vi "Core_[HSMS]Not Selected(Active).vi"(8 "error in (no error)":errorcluster, 11 "HSMS Class in":refnum<class "HSMS Class.lvclass">) -> (0 "error out":errorcluster, 3 "HSMS Class out":refnum<class "HSMS Class.lvclass">)   [LabVIEW 2020, in "SECS Communication.lvlib" / "HSMS Class.lvclass"]
uses:
  HSMS Class.lvclass
  SType.ctl
  Message Packet.ctl
  Message Header.ctl
  PType.ctl
  Notifier Type.ctl
  HSMS Class.lvclass/HSMS Class.ctl
  HSMS State.ctl
  Read Session ID.vi
  Read T6(Control Timeout).vi
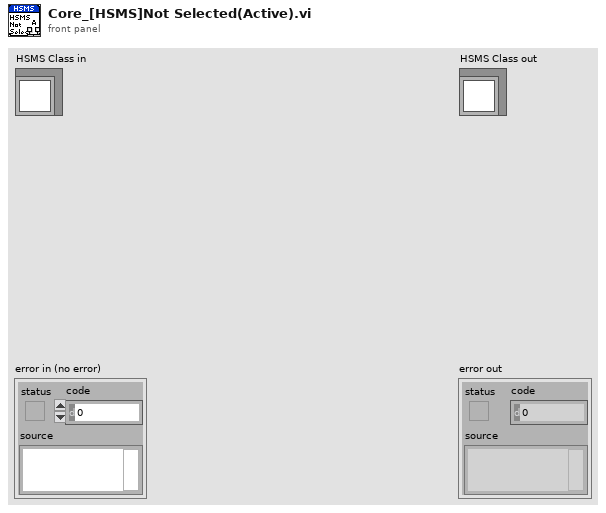
[diagram p1: front panel]
types:
  T1 = typedef "SECS Communication.lvlib/HSMS Class.lvclass/Message Header.ctl" = cluster{"Byte 0-1(Session ID)":u16, "W-Bit":bool, "Byte 2":u8, "Byte 3":u8, "Byte 4(PType)":T2, "Byte 5(SType)":T3, "Byte 6-9(System Btyes)":u8[]}
  T2 = typedef "SECS Communication.lvlib/HSMS Class.lvclass/PType.ctl" = enum8{"SECS-II Encoding", "Reserved"}
  T3 = typedef "SECS Communication.lvlib/HSMS Class.lvclass/SType.ctl" = enum8{"Data Message", "Select.req", "Select.rsp", "Deselect.req", "Deselect.rsp", "Linktest.req", "Linktest.rsp", "Reject.req", "Separate.req"}
  T4 = typedef "SECS Communication.lvlib/HSMS Class.lvclass/Notifier Type.ctl" = enum16{"TCPIP Connect", "TCPIP Disconnect", "Receive Message", "Send Message", "T3 Timeout", "T6 Timeout", "T7 Timeout", "Error", "Stop"}
  T5 = typedef "SECS Communication.lvlib/HSMS Class.lvclass/Message Packet.ctl" = cluster{"Message Header Cluster":T1, "Message Header":u8[], "Message Text":u8[]}
  T6 = typedef "SECS Communication.lvlib/HSMS Class.lvclass/HSMS State.ctl" = enum16{"[TCP/IP]Not Connect", "[HSMS]Not Selected", "[HSMS]Selected", "Stop"}
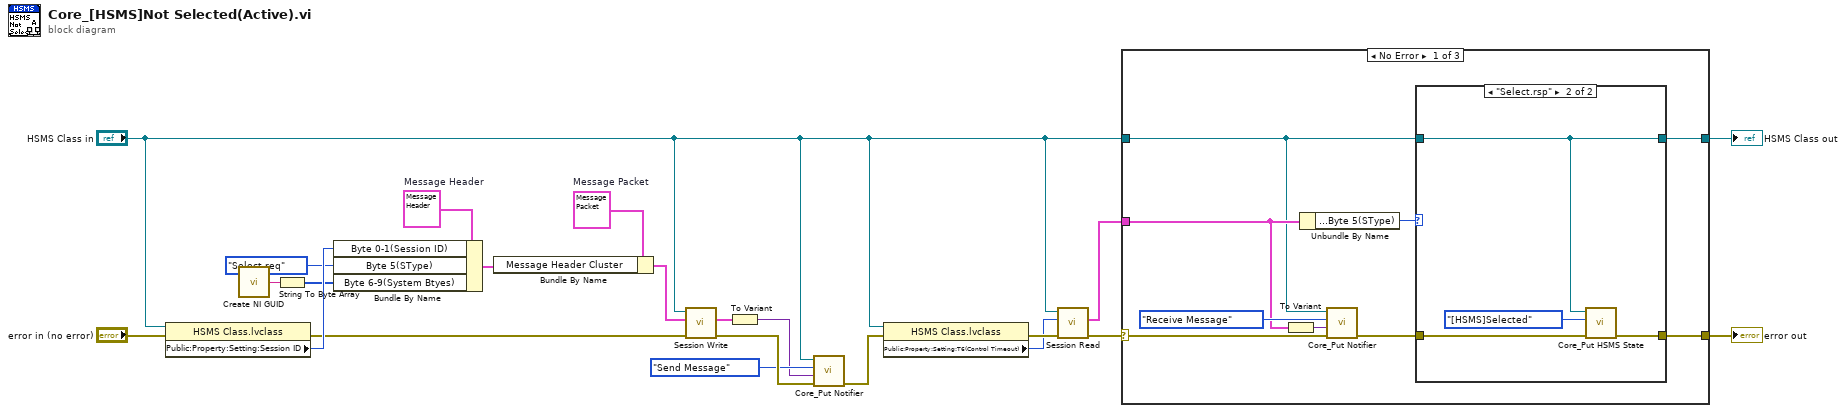
[diagram p0: block diagram]
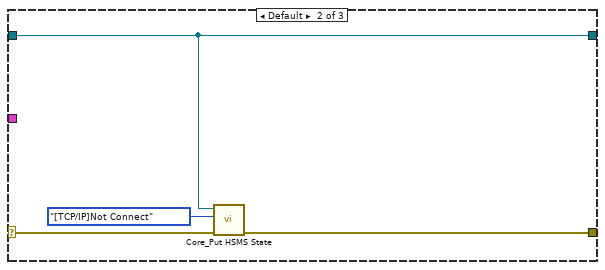
[diagram p3: hidden frame]
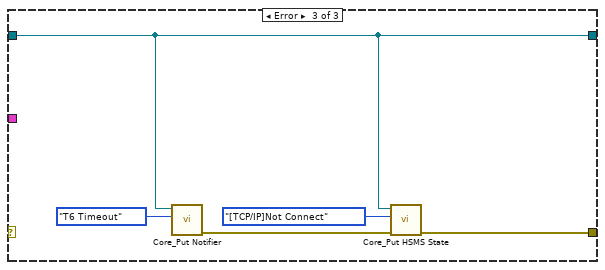
[diagram p4: hidden frame]
diagram:
  w18 = T1 {"Byte 0-1(Session ID)"=0, "W-Bit"=FALSE, "Byte 2"=0, "Byte 3"=0, "Byte 4(PType)"=enum."SECS-II Encoding", "Byte 5(SType)"=enum."Select.req", "Byte 6-9(System Btyes)"=[]}  # Message Header
  w13 = T5 {"Message Header Cluster"={"Byte 0-1(Session ID)"=0, "W-Bit"=FALSE, "Byte 2"=0, "Byte 3"=0, "Byte 4(PType)"=enum."SECS-II Encoding", "Byte 5(SType)"=enum."Data Message", "Byte 6-9(System Btyes)"=[]}, "Message Header"=[], "Message Text"=[]}  # Message Packet
  n1 = property class="HSMS Class.lvclass"(reference="HSMS Class in", error in="error in (no error)") -> (error out=w9:errorcluster, "Public:Property:Setting:Session ID"=w17:u16)  [unwired: 1 out]
  n2 = call <vilib>:"Create NI GUID.vi"() -> ("NI GUID"=w15:string)
  n3 = String To Byte Array(string=w15) -> (unsigned byte array=w14:u8[])
  n4 = Bundle By Name(cluster=w18, "Byte 0-1(Session ID)"=w17, "Byte 5(SType)"=SType."Select.req", "Byte 6-9(System Btyes)"=w14) -> (w12:T1)
  n5 = Bundle By Name(cluster=w13, "Message Header Cluster"=w12) -> (w6:T5)
  n6 = call "Session Write.vi"("error in (no error)"=w9, "Message Packet In"=w6, "HSMS Class in"="HSMS Class in") -> ("error out"=w8:errorcluster, "Message Packet Out"=w1:T5)  [unwired: 6 in, 1 out]
  n7 = To Variant(anything=w1) -> (Variant=w5:variant)
  n8 = call "Core_Put Notifier.vi"("error in (no error)"=w8, "Data"=w5, "Notifier Type"=Notifier_Type."Send Message", "HSMS Class in"="HSMS Class in") -> ("error out"=w4:errorcluster)  [unwired: 6 in, 1 out]
  n9 = property class="HSMS Class.lvclass"(reference="HSMS Class in", error in=w4) -> (error out=w3:errorcluster, "Public:Property:Setting:T6(Control Timeout)"=w2:i32)  [unwired: 1 out]
  n10 = call "Session Read.vi"("error in (no error)"=w3, "Timeout"=w2, "HSMS Class in"="HSMS Class in") -> ("error out"=w10:errorcluster, "Message Packet"=w11:T5)  [unwired: 6 in, 1 out]
  n11 = case shown="No Error" w10 {
    selector: w10 -> [w28 w40 _]
    tunnel: w11 -> [w27 _ _]
    tunnel: [w30 w38 w42] -> w21
    tunnel: "HSMS Class in" -> [w24 w39 w43]
    tunnel: [w23 w39 w43] -> w20
    frame No Error {
      n12 = To Variant(anything=w27) -> (Variant=w26:variant)
      n13 = Unbundle By Name(w27) -> ("Message Header Cluster.Byte 5(SType)"=w25:T3)
      n14 = call "Core_Put Notifier.vi"("error in (no error)"=w28, "Data"=w26, "Notifier Type"=Notifier_Type."Receive Message", "HSMS Class in"=w24) -> ("error out"=w29:errorcluster)  [unwired: 6 in, 1 out]
      n15 = case shown="\"Select.rsp\"" w25 {
        tunnel: w29 -> [w33 w36]
        tunnel: [w33 w34] -> w30
        tunnel: w24 -> [w32 w35]
        tunnel: [w32 w35] -> w23
        frame Default {
        }
        frame "Select.rsp" {
          n16 = call "Core_Put HSMS State.vi"("error in (no error)"=w36, "HSMS State"=HSMS_State."[HSMS]Selected", "HSMS Class in"=w35) -> ("error out"=w34:errorcluster)  [unwired: 7 in, 1 out]
        }
      }
    }
    frame Default {
      n17 = call "Core_Put HSMS State.vi"("error in (no error)"=w40, "HSMS State"=HSMS_State."[TCP/IP]Not Connect", "HSMS Class in"=w39) -> ("error out"=w38:errorcluster)  [unwired: 7 in, 1 out]
    }
    frame Error {
      n18 = call "Core_Put Notifier.vi"("Notifier Type"=Notifier_Type."T6 Timeout", "HSMS Class in"=w43) -> ("error out"=w44:errorcluster)  [unwired: 8 in, 1 out]
      n19 = call "Core_Put HSMS State.vi"("error in (no error)"=w44, "HSMS State"=HSMS_State."[TCP/IP]Not Connect", "HSMS Class in"=w43) -> ("error out"=w42:errorcluster)  [unwired: 7 in, 1 out]
    }
  }
  "error out" <- w21
  "HSMS Class out" <- w20
